vi "NotifyIcon - Register .NET Events Callback.vi"(6 "Events to register":T1[](array[typedef]), 8 "error in (no error)":errorcluster, 10 "NotifyIcon User Event Ref":T2, 11 "NotifyIcon reference in":refnum<k24>) -> (0 "error out":errorcluster, 2 ".NET event refs":refnum<k27>[](array[refnum]), 3 "NotifyIcon reference out":refnum<k24>)   [LabVIEW 2020]
uses:
  System.Windows.Forms
  TypeDefs/NotifyIcon User Event Ref.ctl
  TypeDefs/NotifyIcon Events.ctl
  TypeDefs/NotifyIcon .NET Callback Parameter.ctl
  TypeDefs/NotifyIcon Event Data.ctl
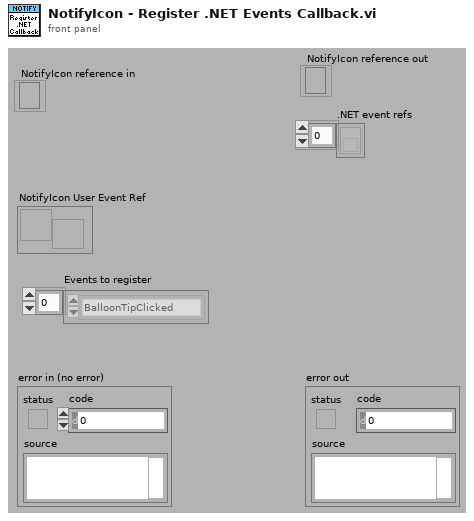
[diagram p1: front panel]
types:
  T1 = typedef "NotifyIcon Events.ctl" = enum16{"BalloonTipClicked", "BalloonTipClosed", "BalloonTipShown", "Click", "Disposed", "DoubleClick", "MouseClick", "MouseDoubleClick", "MouseDown", "MouseMove", "MouseUp", "MenuItemClick", "MenuItemSelect"}
  T2 = typedef "NotifyIcon User Event Ref.ctl" = refnum<user-event>
  T3 = typedef "NotifyIcon .NET Callback Parameter.ctl" = cluster{"NotifyIcon User Event Ref":T2, "Event Data":variant}
  T4 = typedef "NotifyIcon Event Data.ctl" = cluster{"NotifyIcon Event":T1, "Data String":string}
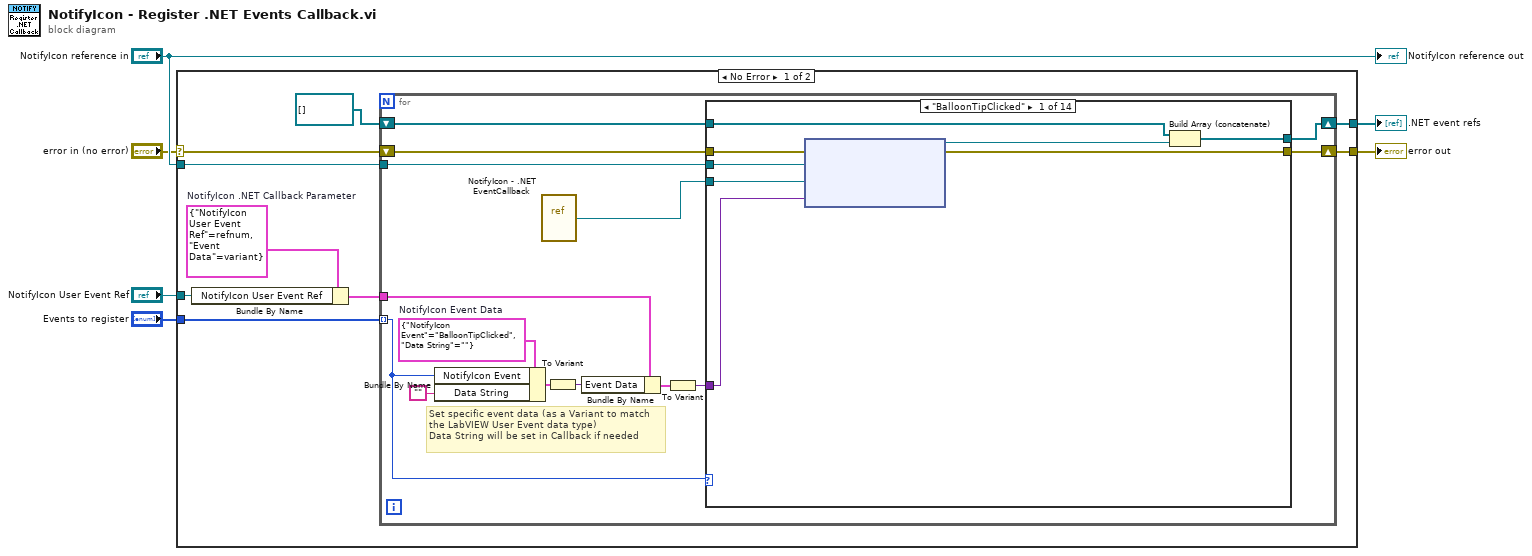
[diagram p0: block diagram]
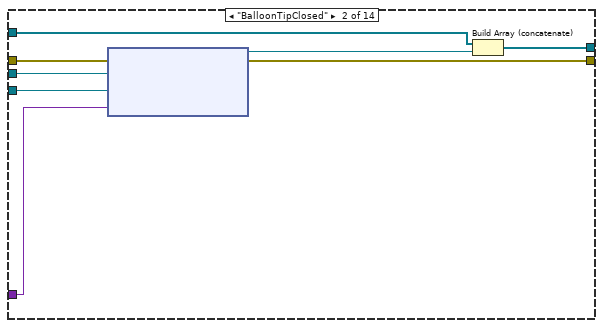
[diagram p2: hidden frame]
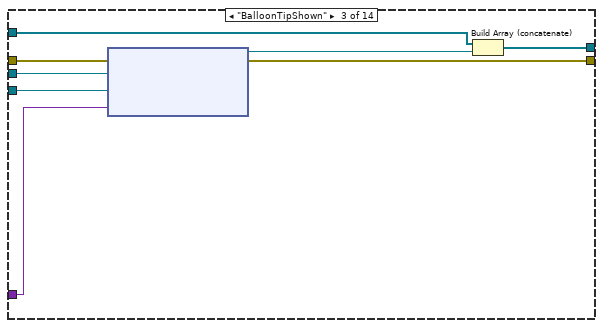
[diagram p3: hidden frame]
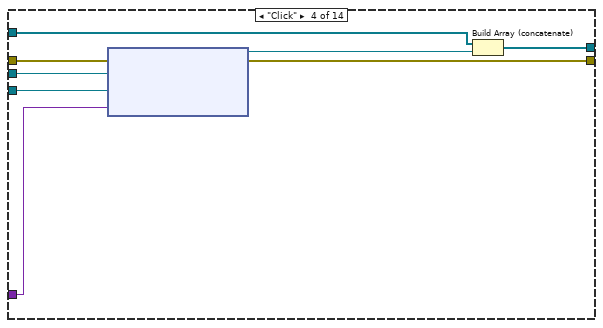
[diagram p4: hidden frame]
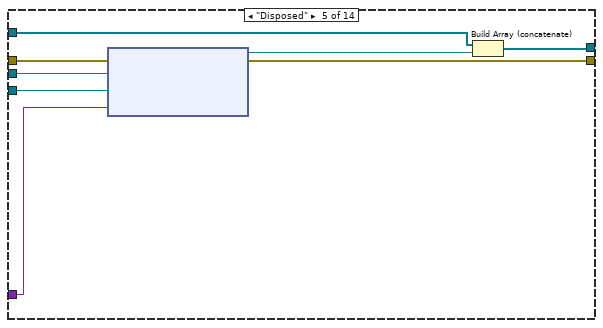
[diagram p5: hidden frame]
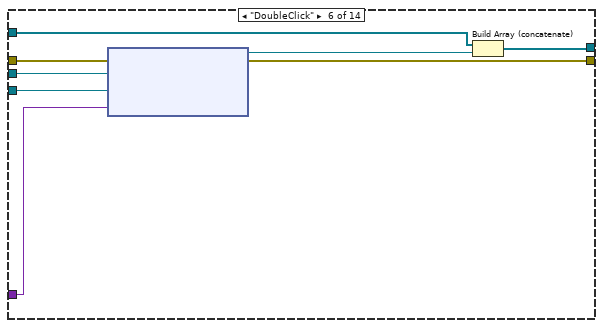
[diagram p6: hidden frame]
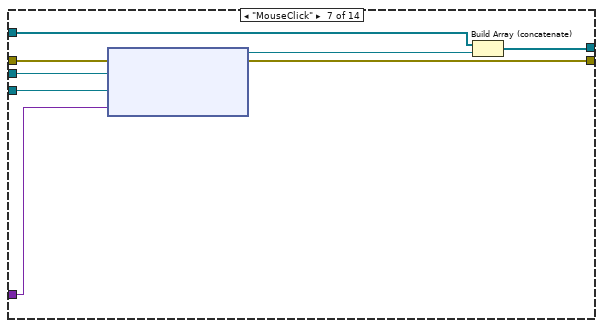
[diagram p7: hidden frame]
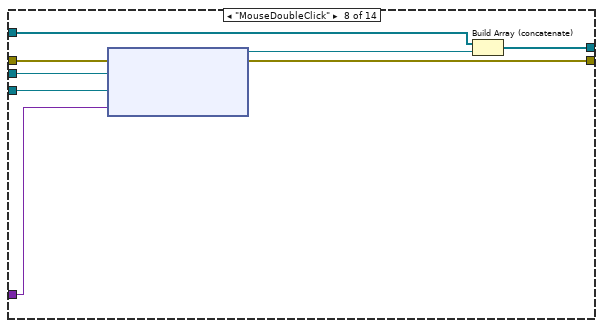
[diagram p8: hidden frame]
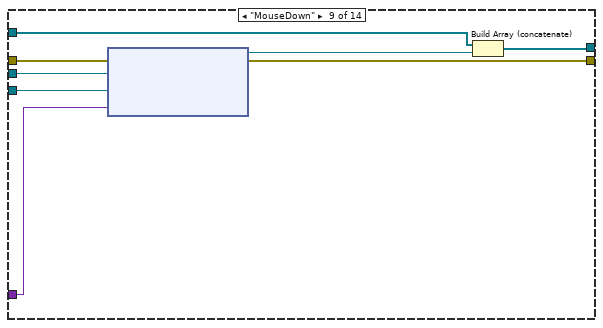
[diagram p9: hidden frame]
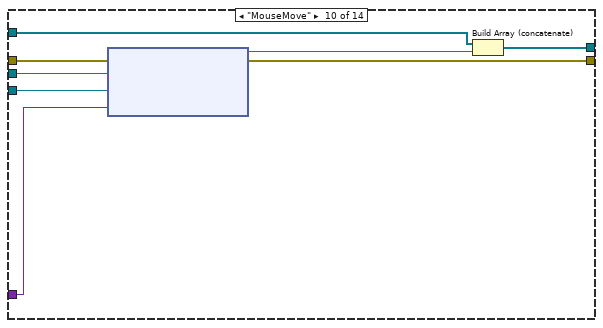
[diagram p10: hidden frame]
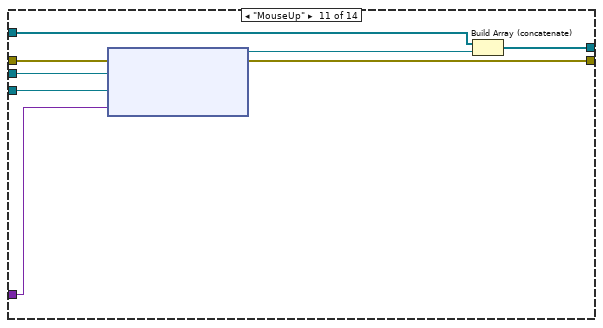
[diagram p11: hidden frame]
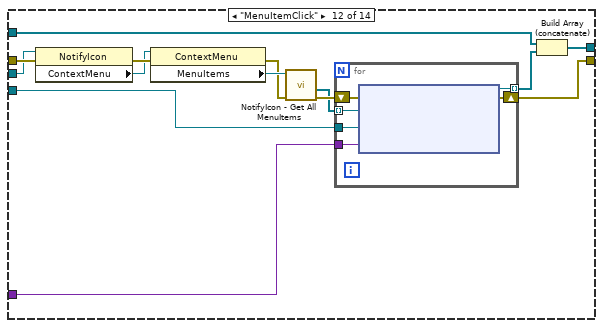
[diagram p12: hidden frame]
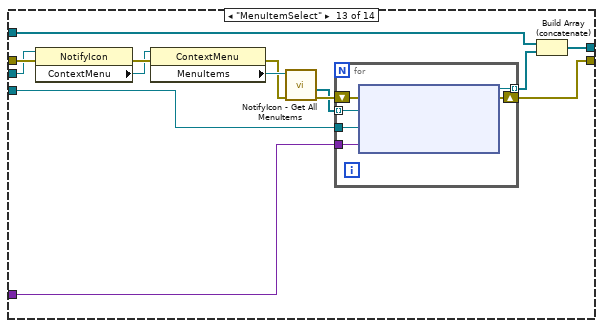
[diagram p13: hidden frame]
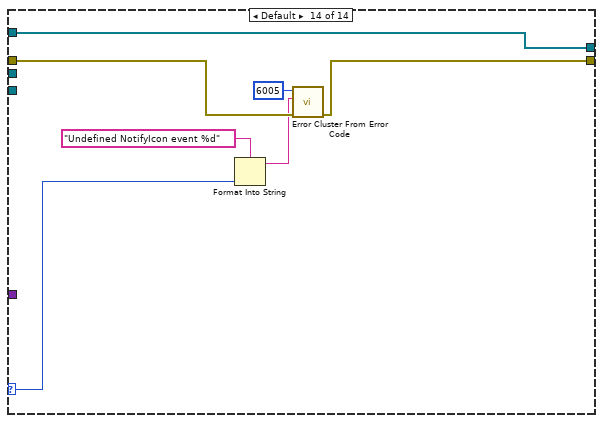
[diagram p14: hidden frame]
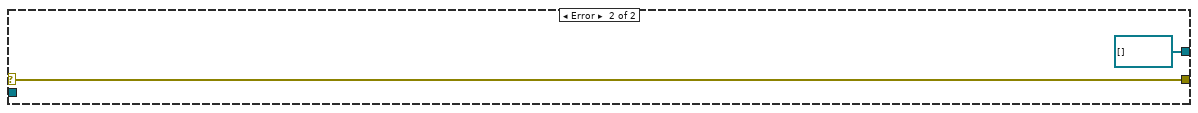
[diagram p15: hidden frame]
diagram:
  n1 = case shown="No Error" "error in (no error)" {
    selector: "error in (no error)" -> [w7 w166]
    tunnel: "NotifyIcon reference in" -> [w15 _]
    tunnel: "NotifyIcon User Event Ref" -> [w13 _]
    tunnel: "Events to register" -> [w12 _]
    tunnel: [w10 w166] -> w3
    tunnel: [w8 refnum<k27>[] []] -> w2
    frame No Error {
      w14 = T3 {"NotifyIcon User Event Ref"=refnum, "Event Data"=variant}  # NotifyIcon .NET Callback Parameter
      n2 = Bundle By Name(cluster=w14, "NotifyIcon User Event Ref"=w13) -> (w11:T3)
      n3 = for {
        tunnel: w15 -> [w29]
        tunnel: w12 -> [w16] mode=indexing
        tunnel: w11 -> [w23]
        shift-right: [w27] -> w10
        shift-left: w7 -> [w28]
        shift-right: [w19] -> w8
        shift-left: refnum<k27>[] [] -> [w18]
        w26 = T4 {"NotifyIcon Event"=enum."BalloonTipClicked", "Data String"=""}  # NotifyIcon Event Data
        # "Set specific event data (as a Variant to match\nthe LabVIEW User Event data type)\nData String will be set in Callback if needed"
        n4 = Bundle By Name(cluster=w26, "NotifyIcon Event"=w16, "Data String"="") -> (w25:T4)
        n5 = vi-ref "NotifyIcon - .NET EventCallback.vi"() -> ("vi reference"=w20:refnum<vi>)
        n6 = To Variant(anything=w25) -> (Variant=w24:variant)
        n7 = Bundle By Name(cluster=w23, "Event Data"=w24) -> (w22:T3)
        n8 = To Variant(anything=w22) -> (Variant=w21:variant)
        n9 = case shown="\"BalloonTipClicked\"" w16 {
          selector: w16 -> [_ _ _ _ _ _ _ _ _ _ _ _ _ w158]
          tunnel: w20 -> [w37 w45 w53 w61 w69 w77 w85 w93 w101 w109 w117 w123 w143 _]
          tunnel: w29 -> [w36 w44 w52 w60 w68 w76 w84 w92 w100 w108 w116 w128 w148 _]
          tunnel: w28 -> [w35 w43 w51 w59 w67 w75 w83 w91 w99 w107 w115 w129 w149 w162]
          tunnel: [w34 w42 w50 w58 w66 w74 w82 w90 w98 w106 w114 w121 w141 w163] -> w27
          tunnel: w21 -> [w33 w41 w49 w57 w65 w73 w81 w89 w97 w105 w113 w122 w142 _]
          tunnel: [w31 w39 w47 w55 w63 w71 w79 w87 w95 w103 w111 w120 w140 w164] -> w19
          tunnel: w18 -> [w30 w38 w46 w54 w62 w70 w78 w86 w94 w102 w110 w119 w138 w164]
          frame "BalloonTipClicked" {
            n10 = node(w35, w36, w37, w33) -> (w32:refnum<k27>, w34:errorcluster)  [unwired: 1 in]
            n11 = Build Array (concatenate)(w30, w32) -> (w31:refnum<k27>[])
          }
          frame "BalloonTipClosed" {
            n12 = node(w43, w44, w45, w41) -> (w40:refnum<k27>, w42:errorcluster)  [unwired: 1 in]
            n13 = Build Array (concatenate)(w38, w40) -> (w39:refnum<k27>[])
          }
          frame "BalloonTipShown" {
            n14 = node(w51, w52, w53, w49) -> (w48:refnum<k27>, w50:errorcluster)  [unwired: 1 in]
            n15 = Build Array (concatenate)(w46, w48) -> (w47:refnum<k27>[])
          }
          frame "Click" {
            n16 = node(w59, w60, w61, w57) -> (w56:refnum<k27>, w58:errorcluster)  [unwired: 1 in]
            n17 = Build Array (concatenate)(w54, w56) -> (w55:refnum<k27>[])
          }
          frame "Disposed" {
            n18 = node(w67, w68, w69, w65) -> (w64:refnum<k27>, w66:errorcluster)  [unwired: 1 in]
            n19 = Build Array (concatenate)(w62, w64) -> (w63:refnum<k27>[])
          }
          frame "DoubleClick" {
            n20 = node(w75, w76, w77, w73) -> (w72:refnum<k27>, w74:errorcluster)  [unwired: 1 in]
            n21 = Build Array (concatenate)(w70, w72) -> (w71:refnum<k27>[])
          }
          frame "MouseClick" {
            n22 = node(w83, w84, w85, w81) -> (w80:refnum<k27>, w82:errorcluster)  [unwired: 1 in]
            n23 = Build Array (concatenate)(w78, w80) -> (w79:refnum<k27>[])
          }
          frame "MouseDoubleClick" {
            n24 = node(w91, w92, w93, w89) -> (w88:refnum<k27>, w90:errorcluster)  [unwired: 1 in]
            n25 = Build Array (concatenate)(w86, w88) -> (w87:refnum<k27>[])
          }
          frame "MouseDown" {
            n26 = node(w99, w100, w101, w97) -> (w96:refnum<k27>, w98:errorcluster)  [unwired: 1 in]
            n27 = Build Array (concatenate)(w94, w96) -> (w95:refnum<k27>[])
          }
          frame "MouseMove" {
            n28 = node(w107, w108, w109, w105) -> (w104:refnum<k27>, w106:errorcluster)  [unwired: 1 in]
            n29 = Build Array (concatenate)(w102, w104) -> (w103:refnum<k27>[])
          }
          frame "MouseUp" {
            n30 = node(w115, w116, w117, w113) -> (w112:refnum<k27>, w114:errorcluster)  [unwired: 1 in]
            n31 = Build Array (concatenate)(w110, w112) -> (w111:refnum<k27>[])
          }
          frame "MenuItemClick" {
            n32 = property class="NotifyIcon"(reference=w128, error in=w129) -> (error out=w131:errorcluster, "ContextMenu"=w130:refnum<k24>)  [unwired: 1 out]
            n33 = property class="ContextMenu"(reference=w130, error in=w131) -> (error out=w126:errorcluster, "MenuItems"=w127:refnum<k24>)  [unwired: 1 out]
            n34 = call "NotifyIcon - Get All MenuItems.vi"("error in (no error)"=w126, "MenuItem Collection reference"=w127) -> ("error out"=w125:errorcluster, "MenuItem references out"=w124:refnum<k24>[])  [unwired: 8 in]
            n35 = for {
              tunnel: w124 -> [w136] mode=indexing
              tunnel: w123 -> [w135]
              tunnel: w122 -> [w134]
              shift-right: [w133] -> w121
              shift-left: w125 -> [w137]
              tunnel: [w132] -> w118 mode=indexing
              n36 = node(w137, w136, w135, w134) -> (w132:refnum<k27>, w133:errorcluster)  [unwired: 1 in]
            }
            n37 = Build Array (concatenate)(w119, w118) -> (w120:refnum<k27>[])
          }
          frame "MenuItemSelect" {
            n38 = property class="NotifyIcon"(reference=w148, error in=w149) -> (error out=w151:errorcluster, "ContextMenu"=w150:refnum<k24>)  [unwired: 1 out]
            n39 = property class="ContextMenu"(reference=w150, error in=w151) -> (error out=w146:errorcluster, "MenuItems"=w147:refnum<k24>)  [unwired: 1 out]
            n40 = call "NotifyIcon - Get All MenuItems.vi"("error in (no error)"=w146, "MenuItem Collection reference"=w147) -> ("error out"=w145:errorcluster, "MenuItem references out"=w144:refnum<k24>[])  [unwired: 8 in]
            n41 = for {
              tunnel: w144 -> [w156] mode=indexing
              tunnel: w143 -> [w155]
              tunnel: w142 -> [w154]
              shift-right: [w153] -> w141
              shift-left: w145 -> [w157]
              tunnel: [w152] -> w139 mode=indexing
              n42 = node(w157, w156, w155, w154) -> (w152:refnum<k27>, w153:errorcluster)  [unwired: 1 in]
            }
            n43 = Build Array (concatenate)(w138, w139) -> (w140:refnum<k27>[])
          }
          frame Default {
            n44 = Format Into String(format string="Undefined NotifyIcon event %d", w158) -> (resulting string=w160:string)  [unwired: 2 in, 1 out]
            n45 = call <vilib>:"Error Cluster From Error Code.vi"("error in (no error)"=w162, "error message (\"\")"=w160, "error code (0)"=6005) -> ("error out"=w163:errorcluster)  [unwired: 6 in]
          }
        }
      }
    }
    frame Error {
    }
  }
  "error out" <- w3
  ".NET event refs" <- w2
  "NotifyIcon reference out" <- "NotifyIcon reference in"
